vi "MAINP Update FaultedFrames.vi"(7 "Controls":refnum<vi>[](array[refnum]), 8 "error in (no error)":errorcluster, 11 "Device Item Ref in":T1 format="%.0x") -> (0 "error out":errorcluster, 3 "Device Item Ref out":T1 format="%.0x")   [LabVIEW 2018, in "CAN Gateway System Explorer.lvlib"]
uses:
  CAN Gateway System Explorer.lvlib
  <vilib>/NI Veristand/Custom Device API/Custom Device Item Ref.ctl
  Types/FramesCluster.ctl
  Shared/Constants.vi
  <vilib>/NI Veristand/Custom Device API/Set Item Property (Variant).vi
  <vilib>/NI Veristand/Custom Device API/Get Item Property (Variant).vi
  <vilib>/NI Veristand/Custom Device API/Custom Device API.lvlib
  Shared/CAN Gateway Shared.lvlib
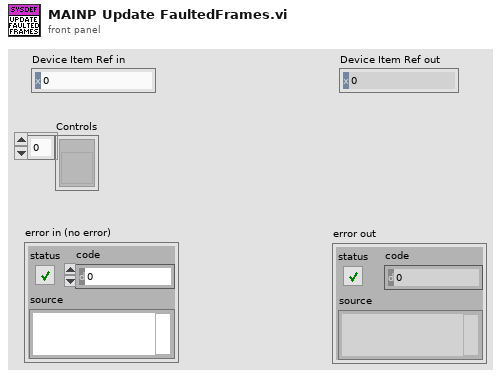
[diagram p1: front panel]
types:
  T1 = typedef "Custom Device API.lvlib/Custom Device Item Ref.ctl" = u64
  T2 = typedef "CAN Gateway System Explorer.lvlib/FramesCluster.ctl" = cluster{"Frame":string, "Fault":bool}
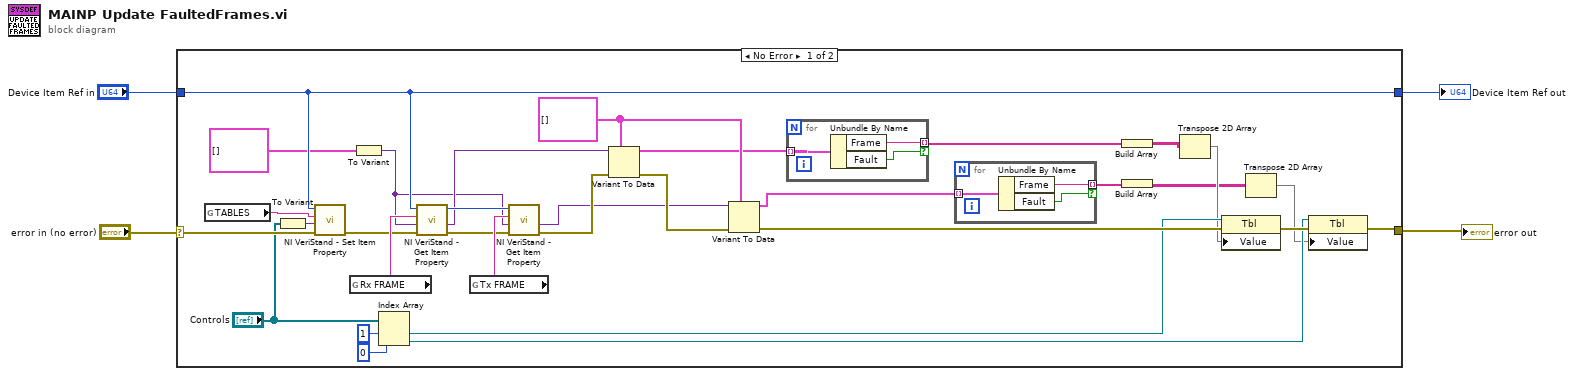
[diagram p0: block diagram]
diagram:
  n1 = case shown="No Error" "error in (no error)" {
    selector: "error in (no error)" -> [w12 w44]
    tunnel: "Device Item Ref in" -> [w10 w43]
    tunnel: [w10 w43] -> w2
    tunnel: [w21 w44] -> w1
    frame No Error {
      w28 = T2[] []
      n2 = global read "Constants.vi" "TABLES"() -> (w7:string)
      n3 = To Variant(anything="Controls") -> (Variant=w9:variant)
      n4 = call-poly <vilib>:"NI VeriStand - Set Item Property.vi"("error in (no error)"=w12, "Value"=w9, "Property Name"=w7, "Item Ref in"=w10) -> ("error out"=w11:errorcluster)  [unwired: 5 in, 2 out]
      n5 = global read "Constants.vi" "Rx FRAME"() -> (w36:string)
      n6 = To Variant(anything=T2[] []) -> (Variant=w5:variant)
      n7 = Index Array(array="Controls", index #1=1 ("index"), index #2=0 ("index")) -> (element #1=w22:refnum<vi>, element #2=w18:refnum<vi>)
      n8 = call-poly <vilib>:"NI VeriStand - Get Item Property.vi"("error in (no error)"=w11, "Default Value"=w5, "Property Name"=w36, "Item Ref in"=w10) -> ("error out"=w33:errorcluster, "Value"=w31:variant, "Item Ref out"=w35:T1)  [unwired: 4 in, 1 out]
      n9 = global read "Constants.vi" "Tx FRAME"() -> (w34:string)
      n10 = call-poly <vilib>:"NI VeriStand - Get Item Property.vi"("error in (no error)"=w33, "Default Value"=w5, "Property Name"=w34, "Item Ref in"=w35) -> ("error out"=w32:errorcluster, "Value"=w29:variant)  [unwired: 4 in, 2 out]
      n11 = Variant To Data(error in=w32, type=w28, Variant=w31) -> (data=w27:T2[], error out=w30:errorcluster)
      n12 = Variant To Data(error in=w30, type=w28, Variant=w29) -> (data=w26:T2[], error out=w23:errorcluster)
      n13 = for {
        tunnel: w27 -> [w42] mode=indexing
        tunnel: [w41] -> w16 mode=indexing if=w40
        n14 = Unbundle By Name(w42) -> ("Frame"=w41:string, "Fault"=w40:bool)
      }
      n15 = for {
        tunnel: w26 -> [w39] mode=indexing
        tunnel: [w38] -> w20 mode=indexing if=w37
        n16 = Unbundle By Name(w39) -> ("Frame"=w38:string, "Fault"=w37:bool)
      }
      n17 = Build Array(w16) -> (w17:string[][])
      n18 = Build Array(w20) -> (w14:string[][])
      n19 = Transpose 2D Array(2D array=w17) -> (transposed array=w15:string[][])
      n20 = property class="Tbl"(reference=w22, error in=w23, "Value"=w15) -> (error out=w19:errorcluster)  [unwired: 1 out]
      n21 = Transpose 2D Array(2D array=w14) -> (transposed array=w13:string[][])
      n22 = property class="Tbl"(reference=w18, error in=w19, "Value"=w13) -> (error out=w21:errorcluster)  [unwired: 1 out]
    }
    frame Error {
    }
  }
  "error out" <- w1
  "Device Item Ref out" <- w2
